vi "Build bars.vi"(6 "Contrast":dbl=1.0, 9 "Draw Area Size":T1, 11 "Bar width (pix)":dbl) -> (3 "bars":picture)   [LabVIEW 2012]
uses:
  <vilib>/Utility/miscctls.llb/LVBoundsTypeDef.ctl
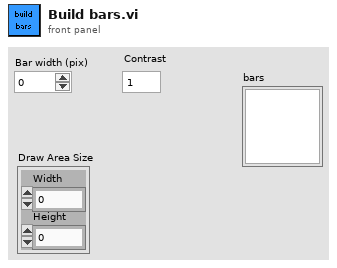
[diagram p1: front panel]
types:
  T1 = typedef "LVBoundsTypeDef.ctl" = cluster{"Width":u32, "Height":u32}
  T2 = cluster{"left":i16, "top":i16, "right":i16, "bottom":i16}
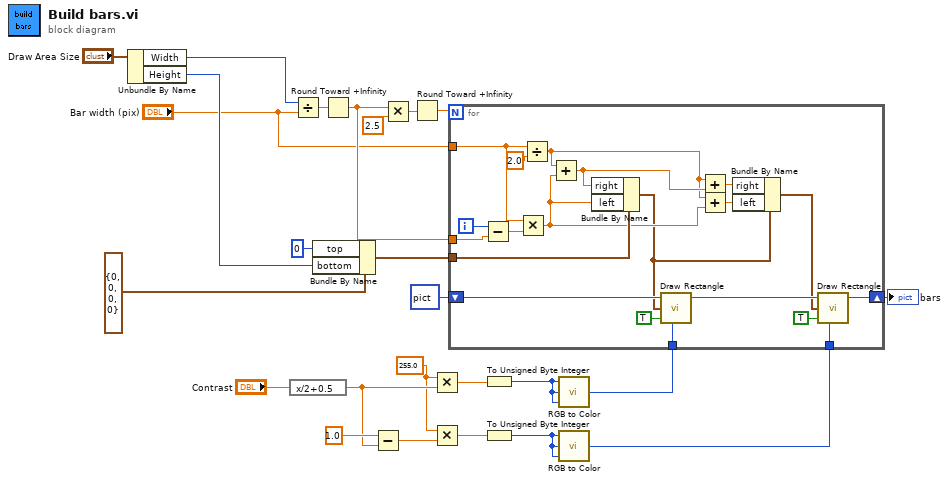
[diagram p0: block diagram]
diagram:
  w5 = 255.0 ("x")
  n1 = Unbundle By Name("Draw Area Size") -> ("Width"=w23:u32, "Height"=w18:u32)
  n2 = expression code="x/2+0.5"("Contrast") -> (w8:dbl)
  n3 = Divide(x=w23, y="Bar width (pix)") -> (x/y=w24:dbl)
  n4 = Bundle By Name(cluster=T2 {"left"=0, "top"=0, "right"=0, "bottom"=0} ("rect"), "top"=i16 0, "bottom"=w18) -> (w17:T2)
  n5 = Round Toward +Infinity(x=w24) -> (ceil(x): smallest int >= x=w21:dbl)
  n6 = Subtract(x=1.0, y=w8) -> (x-y=w6:dbl)
  n7 = Multiply(x=w21, y=2.5) -> (x*y=w16:dbl)
  n8 = Round Toward +Infinity(x=w16) -> (ceil(x): smallest int >= x=w15:dbl)
  n9 = Multiply(x=w5, y=w8) -> (x*y=w7:dbl)
  n10 = Multiply(x=w5, y=w6) -> (x*y=w4:dbl)
  n11 = To Unsigned Byte Integer(number=w7) -> (unsigned 8bit integer=w10:u8)
  n12 = To Unsigned Byte Integer(number=w4) -> (unsigned 8bit integer=w3:u8)
  n13 = call <vilib>:"RGB to Color.vi"("B"=w10, "G"=w10, "R"=w10) -> ("Color"=w12:u32)
  n14 = call <vilib>:"RGB to Color.vi"("B"=w3, "G"=w3, "R"=w3) -> ("Color"=w2:u32)
  n15 = for {
    N: w15 -> [_]
    tunnel: w21 -> [w44]
    tunnel: w17 -> [w42]
    tunnel: "Bar width (pix)" -> [w38]
    shift-right: [w27] -> w14
    shift-left: picture data[5B] ("new picture") -> [w41]
    tunnel: w12 -> [w39]
    tunnel: w2 -> [w26]
    i -> [w45]
    n16 = Subtract(x=w45, y=w44) -> (x-y=w43:dbl)
    n17 = Multiply(x=w38, y=w43) -> (x*y=w35:dbl)
    n18 = Divide(x=w38, y=2.0) -> (x/y=w31:dbl)
    n19 = Add(x=w31, y=w35) -> (x+y=w32:dbl)
    n20 = Bundle By Name(cluster=w42, "right"=w32, "left"=w35) -> (w34:T2)
    n21 = call <vilib>:"Draw Rectangle.vi"("picture"=w41, "rect"=w34, "fill?(F)"=TRUE, "color(black)"=w39) -> ("new picture"=w29:picture)  [unwired: 5 in]
    n22 = Add(x=w31, y=w32) -> (x+y=w33:dbl)
    n23 = Add(x=w31, y=w35) -> (x+y=w36:dbl)
    n24 = Bundle By Name(cluster=w34, "right"=w33, "left"=w36) -> (w28:T2)
    n25 = call <vilib>:"Draw Rectangle.vi"("picture"=w29, "rect"=w28, "fill?(F)"=TRUE, "color(black)"=w26) -> ("new picture"=w27:picture)  [unwired: 5 in]
  }
  "bars" <- w14
